vi "FilterStatus.vi"(0 "VisaCluster":T1, 11 "error in (no error)":errorcluster) -> (4 "VisaCluster":T1, 6 "Display":string, 8 "Answer":string, 10 "Filter":bool, 15 "error out":errorcluster)   [LabVIEW 2014, in "FH 55.lvlib"]
doc: "Diese VI zeigt ob der Filter eingeschaltet oder ausgeschaltet ist.\n\nThis VI shows whether the filter is turned on or turned off."
uses:
  FH 55.lvlib
  TypeDef/VisaCluster.ctl
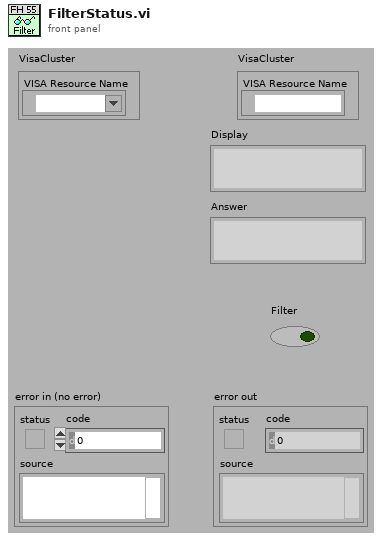
[diagram p1: front panel]
types:
  T1 = typedef "FH 55.lvlib/VisaCluster.ctl" = cluster{"VISA Resource Name":refnum<visa-resource-name>}
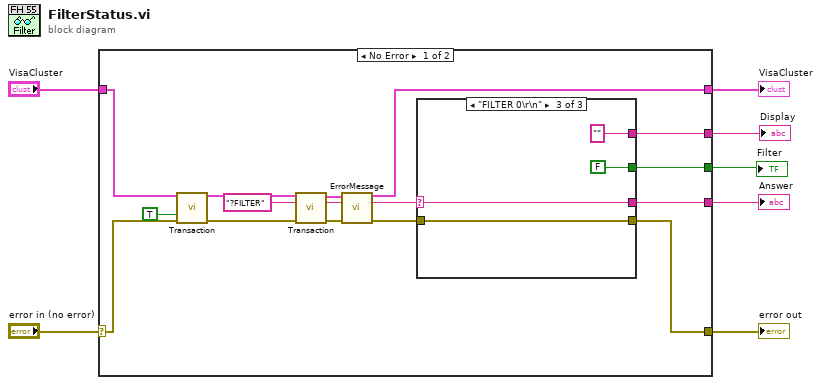
[diagram p0: block diagram]
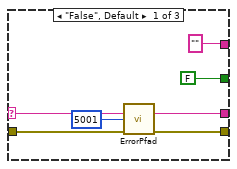
[diagram p2: hidden frame]
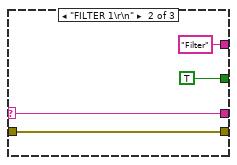
[diagram p3: hidden frame]
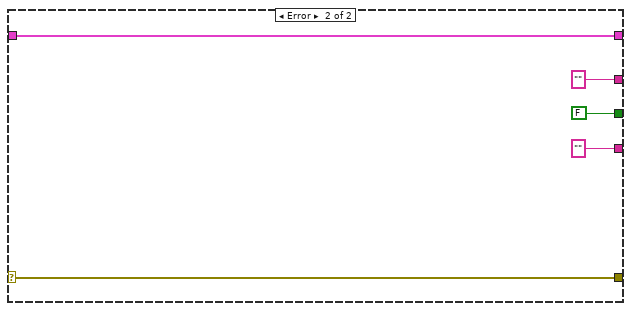
[diagram p4: hidden frame]
diagram:
  n1 = case shown="No Error" "error in (no error)" {
    selector: "error in (no error)" -> [w19 w41]
    tunnel: "VisaCluster" -> [w17 w42]
    tunnel: [w23 w42] -> w3
    tunnel: [w12 w41] -> w5
    tunnel: [w11 ""] -> w4
    tunnel: [w14 FALSE] -> w2
    tunnel: [w8 ""] -> w1
    frame No Error {
      n2 = call "Transaction.vi"("VisaCluster"=w17, "Read Only? (False)"=TRUE, "error in (no error)"=w19) -> ("VisaCluster"=w16:T1, "error out"=w18:errorcluster)  [unwired: 9 in, 2 out]
      n3 = call "Transaction.vi"("VisaCluster"=w16, "Command"="?FILTER", "error in (no error)"=w18) -> ("VisaCluster"=w21:T1, "Answer"=w9:string, "error out"=w22:errorcluster)  [unwired: 9 in, 1 out]
      n4 = call "ErrorMessage.vi"("VisaCluster"=w21, "Message In"=w9, "error in (no error)"=w22) -> ("VisaCluster"=w23:T1, "Message Out"=w10:string, "error out"=w13:errorcluster)  [unwired: 10 in]
      n5 = case shown="\"FILTER 0\\r\\n\"" w10 {
        selector: w10 -> [w25 w31 w36]
        tunnel: [FALSE TRUE FALSE] -> w14
        tunnel: w13 -> [w28 w32 w35]
        tunnel: [w27 w32 w35] -> w12
        tunnel: [w25 w31 w36] -> w11
        tunnel: ["" "Filter" ""] -> w8
        frame "False", Default {
          n6 = call "ErrorPfad.vi"("Message In"=w25, "Numeric"=5001, "error in (no error)"=w28) -> ("error out"=w27:errorcluster)  [unwired: 11 in, 1 out]
        }
        frame "FILTER 1\r\n" {
        }
        frame "FILTER 0\r\n" {
        }
      }
    }
    frame Error {
    }
  }
  "error out" <- w5
  "Answer" <- w4
  "VisaCluster" <- w3
  "Filter" <- w2
  "Display" <- w1
